vi "Process Diff Images.vi"(8 "error in (no error)":errorcluster, 11 "Report path":path) -> (0 "error out":errorcluster)   [LabVIEW 2020, in "Graphical Diff.lvlib"]
uses:
  Graphical Diff.lvlib
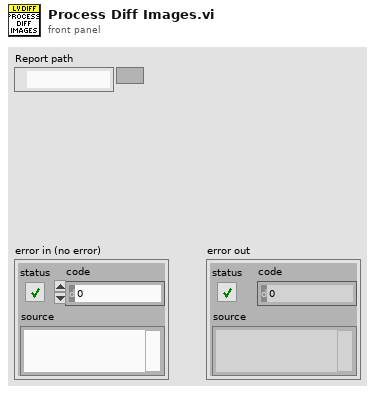
[diagram p1: front panel]
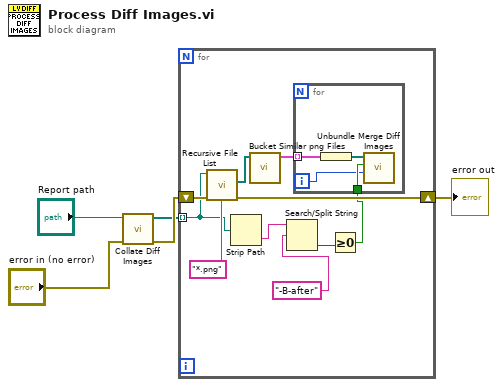
[diagram p0: block diagram]
diagram:
  n1 = call "Collate Diff Images.vi"("error in (no error)"="error in (no error)", "Report XML Path"="Report path") -> ("error out"=w4:errorcluster, "Collated Directories"=w1:path[])  [unwired: 8 in]
  n2 = for {
    shift-right: [w12] -> w5
    shift-left: w4 -> [w13]
    tunnel: w1 -> [w10] mode=indexing
    n3 = call <vilib>:"Recursive File List.vi"("pattern"="*.png", "error in (no error)"=w13, "Folder Path"=w10) -> ("error out"=w12:errorcluster, "All Files in Dir"=w15:path[])  [unwired: 4 in, 3 out]
    n4 = Strip Path(path=w10) -> (name=w9:string)  [unwired: 1 out]
    n5 = call "Bucket Similar png Files.vi"("All PNG Files"=w15) -> ("All PNG Files (Bucketed by Near-Matches)"=w14:cluster{"Similar PNG Files":path[]}[])  [unwired: 9 in]
    n6 = Search/Split String(string=w9, search string/char (-)="-B-after" ("pattern")) -> (offset of match=w7:i32)  [unwired: 1 in, 2 out]
    n7 = Greater Or Equal To 0?(x=w7) -> (x >= 0?=w6:bool)
    n8 = for {
      tunnel: w14 -> [w19] mode=indexing
      tunnel: w6 -> [w17]
      i -> [w16]
      n9 = Unbundle(w19) -> ("Similar PNG Files"=w18:path[])
      n10 = call "Merge Diff Images.vi"("ID"=w16, "Before = F | After = T?"=w17, "Diff PNG Files"=w18) -> ()  [unwired: 8 in]
    }
  }
  "error out" <- w5
